vi "C37 Create Error Message.vi"(6 "VI Reference":refnum<vi>, 8 "error in (no error)":errorcluster, 10 "Error Messages":string[](array[string]), 11 "function return":i32) -> (0 "error out":errorcluster)   [LabVIEW 2018, in "S3DK.lvlib" / "C37118-DLL.lvlib"]
uses:
  C37118-DLL.lvlib
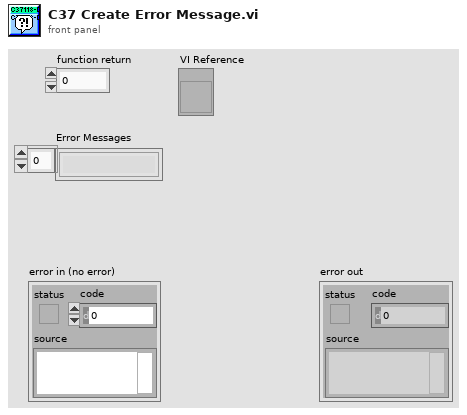
[diagram p1: front panel]
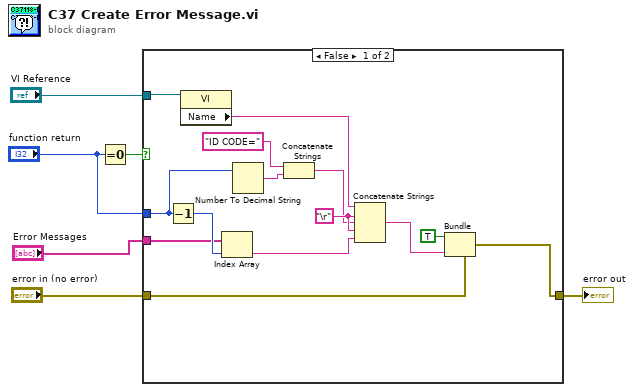
[diagram p0: block diagram]
diagram:
  n1 = Equal To 0?(x="function return") -> (x = 0?=w6:bool)
  n2 = case shown="False" w6 {
    tunnel: "VI Reference" -> [w20 _]
    tunnel: "function return" -> [w10 _]
    tunnel: "error in (no error)" -> [w17 w21]
    tunnel: [w13 w21] -> w2
    tunnel: "Error Messages" -> [w18 _]
    frame False {
      w11 = "\r"
      n3 = Decrement(x=w10) -> (x-1=w19:i32)
      n4 = property class="VI"(reference=w20) -> ("Name"=w16:string)  [unwired: 1 in, 2 out]
      n5 = Index Array(array=w18, index=w19) -> (element=w12:string)
      n6 = Number To Decimal String(number=w10) -> (decimal integer string=w8:string)  [unwired: 1 in]
      n7 = Concatenate Strings("ID CODE=" ("string"), w8) -> (w7:string)
      n8 = Concatenate Strings(w16, w11, w7, w11, w12) -> (w15:string)
      n9 = Bundle(cluster=w17, "status"=TRUE, "source"=w15) -> (w13:errorcluster)  [unwired: 1 in]
    }
    frame True {
    }
  }
  "error out" <- w2
